vi "AI 20K Vibration.vi"(8 "error in (no error)":errorcluster, 11 "All Queue":T2) -> (0 "error out":errorcluster)   [LabVIEW 2022 SP3]
uses:
  Controls/ALL Health.ctl
  6D_Global.vi
  <vilib>/DAQmx/create/channels.llb/DAQmx Create Channel (AI-Voltage-Basic).vi
  <vilib>/DAQmx/create/scale.llb/DAQmx Create Scale (Map Ranges).vi
  <vilib>/DAQmx/configure/timing.llb/DAQmx Timing (Sample Clock).vi
  <vilib>/DAQmx/configure/trigger.llb/DAQmx Start Trigger (Time).vi
  <vilib>/DAQmx/read.llb/DAQmx Read (Analog 1D Wfm NChan NSamp).vi
  <vilib>/Utility/error.llb/DialogType.ctl
  Controls/All Queue Ref.ctl
panel:
  in  "AI Config":T1(array[cluster])=[{"AI signal Lists"="D_PT_1", "AI Channel List"="cDAQ9185-1E540F5Mod4/ai4", "Prescale Min"=0.0, "Prescale Max"=10.0, "Sensor Min"=0.0, "Sensor Max"=60.0, "Units"="bar"}, {"AI signal Lists"="D_PT_2", "AI Channel List"="cDAQ9185-1E540F5Mod4/ai7", "Prescale Min"=0.0, "Prescale Max"=10.0, "Sensor Min"=0.0, "Sensor Max"=60.0, "Units"="bar"}, {"AI signal Lists"="M_PT_1", "AI Channel List"="cDAQ9185-1E540F5Mod4/ai0", "Prescale Min"=0.0, "Prescale Max"=10.0, "Sensor Min"=0.0, "Sensor Max"=60.0, "Units"="bar"}, {"AI signal Lists"="M_PT_2", "AI Channel List"="cDAQ9185-1E540F5Mod4/ai9", "Prescale Min"=0.0, "Prescale Max"=10.0, "Sensor Min"=0.0, "Sensor Max"=60.0, "Units"="bar"}, {"AI signal Lists"="M_PT_3", "AI Channel List"="cDAQ9185-1E540F5Mod4/ai10", "Prescale Min"=0.0, "Prescale Max"=10.0, "Sensor Min"=0.0, "Sensor Max"=60.0, "Units"="bar"}, {"AI signal Lists"="D_RTD_1", "AI Channel List"="cDAQ9185-1E540F5Mod4/ai5", "Prescale Min"=0.0, "Prescale Max"=10.0, "Sensor Min"=73.0, "Sensor Max"=573.0, "Units"="k"}, {"AI signal Lists"="D_RTD_2", "AI Channel List"="cDAQ9185-1E540F5Mod4/ai6", "Prescale Min"=0.0, "Prescale Max"=10.0, "Sensor Min"=73.0, "Sensor Max"=573.0, "Units"="k"}, {"AI signal Lists"="M_RTD_1", "AI Channel List"="cDAQ9185-1E540F5Mod4/ai1", "Prescale Min"=0.0, "Prescale Max"=10.0, "Sensor Min"=73.0, "Sensor Max"=573.0, "Units"="k"}, {"AI signal Lists"="M_RTD_2", "AI Channel List"="cDAQ9185-1E540F5Mod4/ai3", "Prescale Min"=0.0, "Prescale Max"=10.0, "Sensor Min"=73.0, "Sensor Max"=573.0, "Units"="k"}, {"AI signal Lists"="M_RTD_3", "AI Channel List"="cDAQ9185-1E540F5Mod4/ai2", "Prescale Min"=0.0, "Prescale Max"=10.0, "Sensor Min"=73.0, "Sensor Max"=573.0, "Units"="k"}]
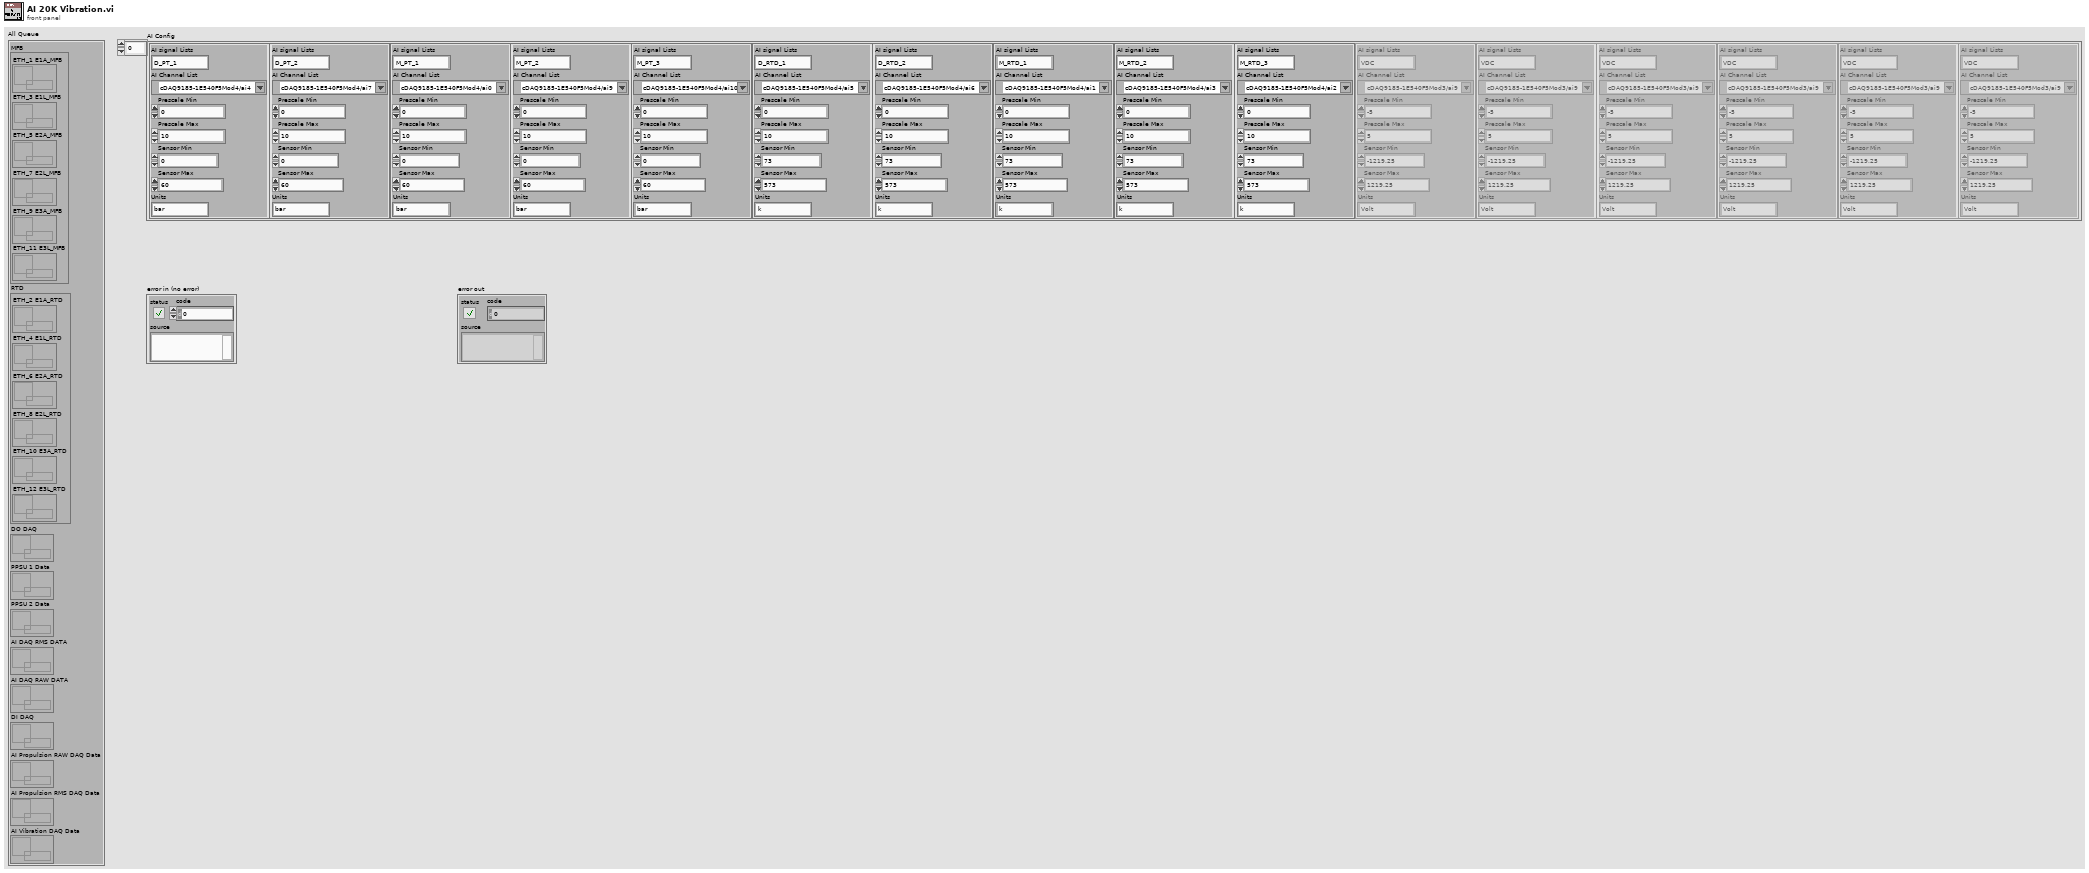
[diagram p1: front panel]
types:
  T1 = cluster{"AI signal Lists":string, "AI Channel List":tag, "Prescale Min":dbl, "Prescale Max":dbl, "Sensor Min":dbl, "Sensor Max":dbl, "Units":string}[]
  T2 = typedef "All Queue Ref.ctl" = cluster{"MFB":cluster{"ETH_1 E1A_MFB":refnum<queue>, "ETH_3 E1L_MFB":refnum<queue>, "ETH_5 E2A_MFB":refnum<queue>, "ETH_7 E2L_MFB":refnum<queue>, "ETH_9 E3A_MFB":refnum<queue>, "ETH_11 E3L_MFB":refnum<queue>}, "RTD":cluster{"ETH_2 E1A_RTD ":refnum<queue>, "ETH_4 E1L_RTD ":refnum<queue>, "ETH_6 E2A_RTD ":refnum<queue>, "ETH_8 E2L_RTD ":refnum<queue>, "ETH_10 E3A_RTD ":refnum<queue>, "ETH_12 E3L_RTD ":refnum<queue>}, "DO DAQ":refnum<queue>, "PPSU 1 Data":refnum<queue>, "PPSU 2 Data":refnum<queue>, "AI DAQ RMS DATA":refnum<queue>, "AI DAQ RAW DATA":refnum<queue>, "DI DAQ":refnum<queue>, "AI Propulsion RAW DAQ Data":refnum<queue>, "AI Propulsion RMS DAQ Data":refnum<queue>, "AI Vibration DAQ Data":refnum<queue>}
  T3 = enum16{"Channel Data Input", "Sampling Data Input", "Read Data", "Stop DAQ"}
  T4 = typedef "ALL Health.ctl" = enum16{"AI HS", "AI Vibration HS", "AI Propulsion HS", "DO HS", "Datalog HS", "PPSU HS", "ETH_1 DAQ", "ETH_1 RTD", "ETH_2 DAQ", "ETH_2 RTD", "ETH_5 RTD"}
  T5 = enum16{"Init", "Read 'All'", "Read 'n'", "Read '1'", "Write '1'", "Write 'n'", "Write 'All'"}
  T6 = cluster{"Samples per channel":i32, "Sampling Rate":dbl, "Sample Mode":i32, "Source":tag}
  T7 = typedef "DialogType.ctl" = u16
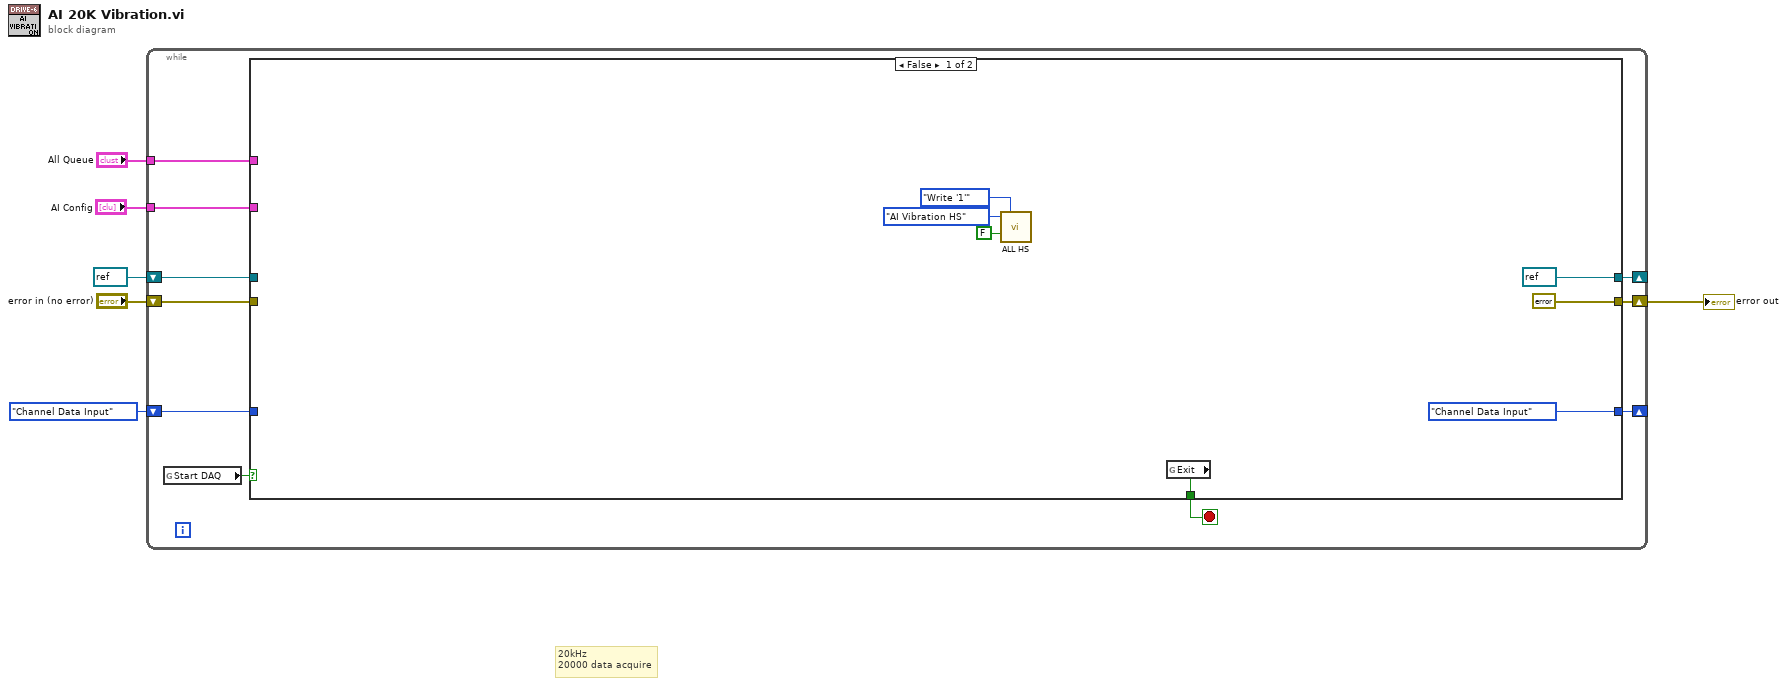
[diagram p0: block diagram]
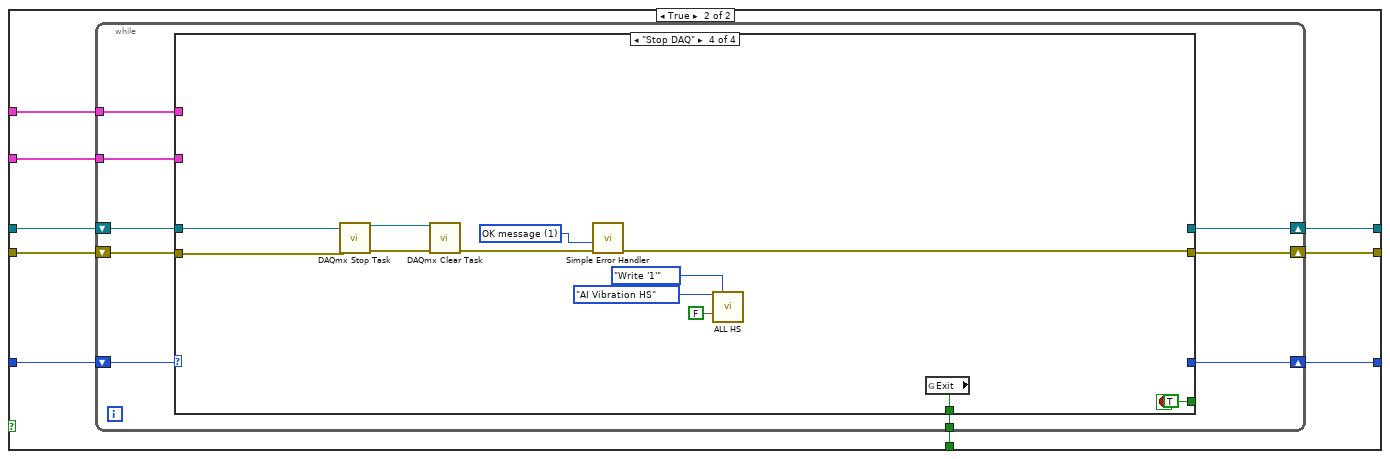
[diagram p2: hidden frame]
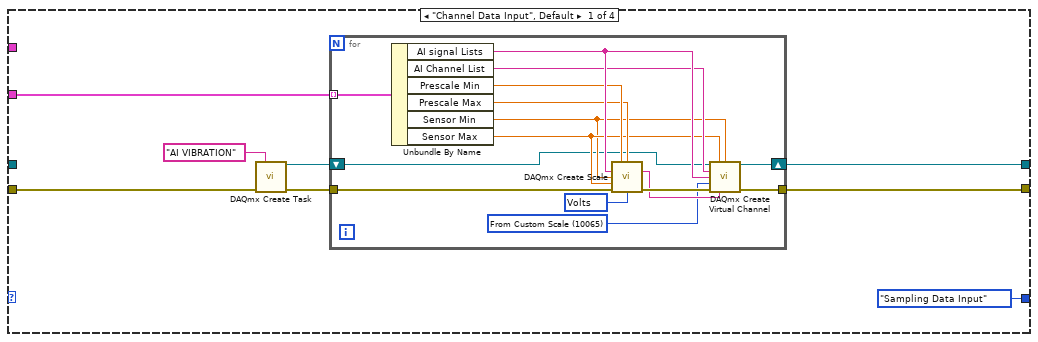
[diagram p3: hidden frame]
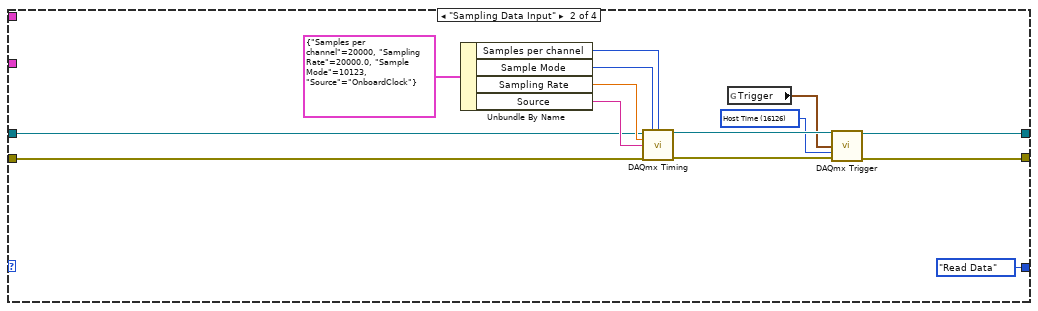
[diagram p4: hidden frame]
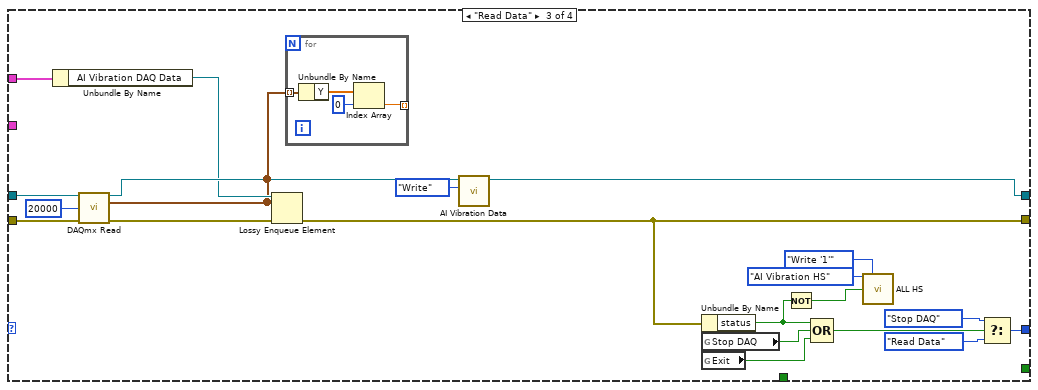
[diagram p5: hidden frame]
diagram:
  # "20kHz \n20000 data acquire"
  n1 = while {
    shift-right: [w13] -> _
    shift-left: T3."Channel Data Input" -> [w16]
    shift-right: [w15] -> _
    shift-left: refnum<k21> refnum ("task out") -> [w14]
    shift-right: [w10] -> w2
    shift-left: "error in (no error)" -> [w11]
    tunnel: "All Queue" -> [w9]
    tunnel: "AI Config" -> [w7]
    stop <- w12 stop-if-true
    n2 = global read "6D_Global.vi" "Start DAQ"() -> (w8:bool)
    n3 = case shown="False" w8 {
      tunnel: w16 -> [_ w32]
      tunnel: [refnum<k21> refnum ("task out") w31] -> w15
      tunnel: w14 -> [_ w30]
      tunnel: [T3."Channel Data Input" w29] -> w13
      tunnel: [w21 w28] -> w12
      tunnel: w11 -> [_ w27]
      tunnel: [errorcluster {"status"=FALSE, "code"=0, "source"=""} ("error out") w25] -> w10
      tunnel: w9 -> [_ w26]
      tunnel: w7 -> [_ w24]
      frame False {
        n4 = call "ALL HS.vi"("Loop"=ALL_Health."AI Vibration HS", "Option"=T5."Write '1'", "Status"=FALSE) -> ()  [unwired: 10 in, 3 out]
        n5 = global read "6D_Global.vi" "Exit"() -> (w21:bool)
      }
      frame True {
        n6 = while {
          tunnel: [w38] -> w28
          tunnel: w26 -> [w36]
          shift-right: [w39] -> w29
          shift-left: w32 -> [w42]
          shift-right: [w41] -> w31
          shift-left: w30 -> [w40]
          shift-right: [w35] -> w25
          shift-left: w27 -> [w37]
          tunnel: w24 -> [w33]
          stop <- w34 stop-if-true
          n7 = case shown="\"Stop DAQ\"" w42 {
            tunnel: w37 -> [w44 w73 w94 w115]
            tunnel: [w45 w69 w84 w105] -> w35
            tunnel: [w47 w70 w96 _] -> w41
            tunnel: w40 -> [_ w75 w95 w113]
            tunnel: [T3."Sampling Data Input" T3."Read Data" w97 _] -> w39
            tunnel: [_ _ _ w111] -> w38
            tunnel: w36 -> [_ _ w86 _]
            tunnel: [_ _ _ TRUE] -> w34
            tunnel: w33 -> [w43 _ _ _]
            frame "Channel Data Input", Default {
              n8 = call <vilib>:"DAQmx Create Task.vi"("new task name"="AI VIBRATION", "error in"=w44) -> ("task out"=w50:refnum<k21>, "error out"=w49:errorcluster)  [unwired: 12 in]
              n9 = for {
                tunnel: w49 -> [w65]
                tunnel: w43 -> [w63] mode=indexing
                shift-right: [w53] -> w47
                shift-left: w50 -> [w52]
                tunnel: [w51] -> w45
                w54 = 10065 items=["Volts"=10348, "From Custom Scale"=10065] ("units")
                w55 = 10348 items=["Volts"=10348, "Amps"=10342, "Deg F"=10144, "Deg C"=10143, "Deg R"=10145, "Kelvins"=10325, "Strain"=10299, "Ohms"=10384, "Hz"=10373, "Seconds"=10364, "Meters"=10219, "Inches"=10379, "Degrees"=10146, "Radians"=10273, "Ticks"=10304, "g"=10186, "m/s^2"=12470, "m/s"=15959, "in/s"=15960, "Pascals"=10081, "Newtons"=15875, "Pounds"=15876, "kgf"=15877, "psi"=15879, "bar"=15880, "Nm"=15881, "oz-in"=15882, "lb-in"=15883, "lb-ft"=15884, "Volts/Volt"=15896, "mVolts/Volt"=15897, "pCoulombs"=16103, "Coulombs"=16102, "From TEDS"=12516] ("pre-scaled units")
                n10 = Unbundle By Name(w63) -> ("AI signal Lists"=w62:string, "AI Channel List"=w61:tag, "Prescale Min"=w59:dbl, "Prescale Max"=w58:dbl, "Sensor Min"=w56:dbl, "Sensor Max"=w57:dbl)
                n11 = call-poly <vilib>:"DAQmx Create Scale.vi"("pre-scaled minimum"=w59, "pre-scaled maximum"=w58, "name"=w62, "scaled minimum"=w56, "scaled maximum"=w57, "error in"=w65, "pre-scaled units"=w55) -> ("scale out"=w60:tag, "error out"=w64:errorcluster)  [unwired: 7 in]
                n12 = call-poly <vilib>:"DAQmx Create Virtual Channel.vi"("task in"=w52, "maximum value"=w57, "minimum value"=w56, "physical channels"=w61, "name to assign"=w62, "units"=w54, "error in"=w64, "custom scale name"=w60) -> ("task out"=w53:refnum<k21>, "error out"=w51:errorcluster)  [unwired: 6 in]
              }
            }
            frame "Sampling Data Input" {
              w68 = 16126 items=["Host Time"=16126, "I/O Device Time"=16127] ("timescale")
              n13 = Unbundle By Name(T6 {"Samples per channel"=20000, "Sampling Rate"=20000.0, "Sample Mode"=10123, "Source"="OnboardClock"} ("Analog Input Samples Data")) -> ("Samples per channel"=w76:i32, "Sample Mode"=w77:i32, "Sampling Rate"=w78:dbl, "Source"=w79:tag)
              n14 = call-poly <vilib>:"DAQmx Timing.vi"("task/channels in"=w75, "sample mode"=w77, "samples per channel"=w76, "rate"=w78, "source"=w79, "error in"=w73) -> ("task out"=w72:refnum<k21>, "error out"=w71:errorcluster)  [unwired: 8 in]
              n15 = global read "6D_Global.vi" "Trigger"() -> (w67:timestamp)
              n16 = call-poly <vilib>:"DAQmx Trigger.vi"("task/channels in"=w72, "when"=w67, "timescale"=w68, "error in"=w71) -> ("task out"=w70:refnum<k21>, "error out"=w69:errorcluster)  [unwired: 10 in]
            }
            frame "Read Data" {
              n17 = Unbundle By Name(w86) -> ("AI Vibration DAQ Data"=w83:refnum<queue>)
              n18 = call-poly <vilib>:"DAQmx Read.vi"("task/channels in"=w95, "number of samples per channel"=20000, "error in"=w94) -> ("task out"=w96:refnum<k21>, "data"=w82:waveform(dbl)[], "error out"=w85:errorcluster)  [unwired: 10 in]
              n19 = Lossy Enqueue Element(queue=w83, element=w82, error in (no error)=w85) -> (error out=w84:errorcluster)  [unwired: 3 out]
              n20 = for {
                tunnel: w82 -> [w101] mode=indexing
                tunnel: [w100] -> _ mode=indexing
                n21 = Unbundle By Name(w101) -> ("Y"=w102:dbl[])
                n22 = Index Array(array=w102, index=0) -> (element=w100:dbl)
              }
              n23 = call "AI Vibration Data.vi"("Enum"=enum16{"Read", "Write"}."Write", "Vibration Data"=w82) -> ()  [unwired: 9 in, 1 out]
              n24 = Unbundle By Name(w84) -> ("status"=w88:bool)
              n25 = global read "6D_Global.vi" "Stop DAQ"() -> (w91:bool)
              n26 = global read "6D_Global.vi" "Exit"() -> (w92:bool)
              n27 = Not(x=w88) -> (.not. x?=w89:bool)
              n28 = Compound Arithmetic op=OR(w88, w91, w92) -> (w87:bool)
              n29 = call "ALL HS.vi"("Loop"=ALL_Health."AI Vibration HS", "Option"=T5."Write '1'", "Status"=w89) -> ()  [unwired: 10 in, 3 out]
              n30 = Select(t=T3."Stop DAQ", s=w87, f=T3."Read Data") -> (s? t:f=w97:T3)
            }
            frame "Stop DAQ" {
              w110 = T7 1 items=["no dialog", "OK message", "continue or stop message", "OK message + warnings", "continue/stop + warnings"] ("type of dialog (OK msg:1)")
              n31 = call <vilib>:"DAQmx Stop Task.vi"("task/channels in"=w113, "error in"=w115) -> ("task out"=w112:refnum<k21>, "error out"=w114:errorcluster)  [unwired: 12 in]
              n32 = call <vilib>:"DAQmx Clear Task.vi"("task in"=w112, "error in"=w114) -> ("error out"=w109:errorcluster)  [unwired: 13 in]
              n33 = call <vilib>:"Simple Error Handler.vi"("type of dialog (OK msg:1)"=w110, "error in (no error)"=w109) -> ("error out"=w105:errorcluster)  [unwired: 3 in, 4 out]
              n34 = call "ALL HS.vi"("Loop"=ALL_Health."AI Vibration HS", "Option"=T5."Write '1'", "Status"=FALSE) -> ()  [unwired: 10 in, 3 out]
              n35 = global read "6D_Global.vi" "Exit"() -> (w111:bool)
            }
          }
        }
      }
    }
  }
  "error out" <- w2
